vi "FileSync_Configure.vi"(8 "error in (no error)":errorcluster, 10 "Dir":path, 11 "Protocol in":refnum<class "Protocol.lvclass">) -> (0 "error out":errorcluster, 3 "Protocol out":refnum<class "Protocol.lvclass">)   [LabVIEW 2020, in "CSM-FileSync.lvlib" / "Protocol.lvclass"]
uses:
  Protocol.lvclass
  Protocol.lvclass/Protocol.ctl
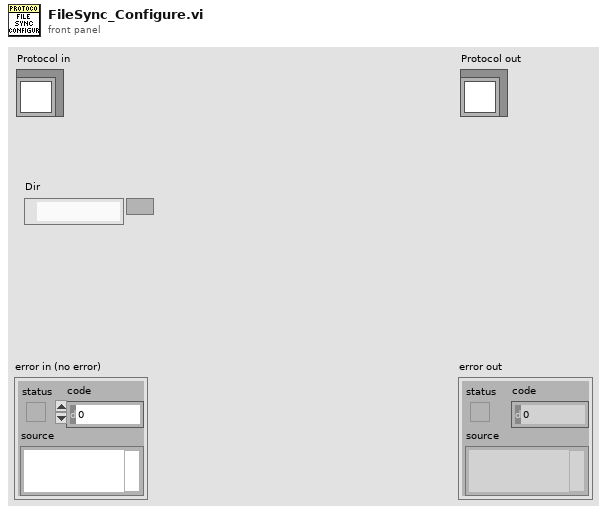
[diagram p1: front panel]
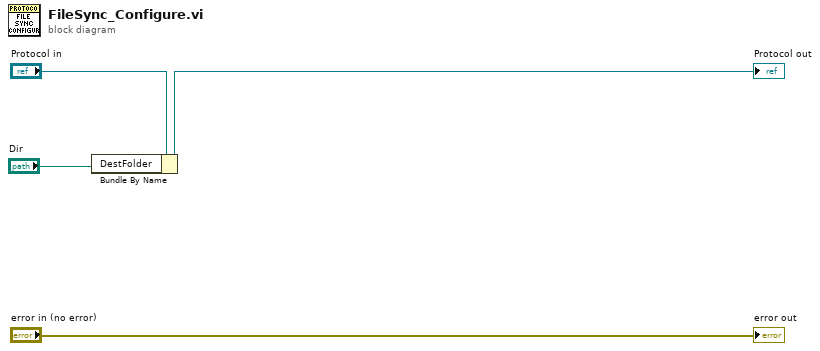
[diagram p0: block diagram]
diagram:
  n1 = Bundle By Name(cluster="Protocol in", "DestFolder"="Dir") -> (→"Protocol out":refnum<class "Protocol.lvclass">)
  "error out" <- "error in (no error)"
